vi "WFS Set Calc Spots To User Reference.vi"(7 "Array Ref Pos Y":u32, 8 "error in (no error)":errorcluster {"code" format="%.0x"}, 9 "Array Ref Pos X":u32, 10 "Reference Type (Relative)":i32(ring) items=["Relative", "Absolute"], 11 "instrument handle":refnum<visa-resource-name>) -> (0 "error out":errorcluster {"code" format="%.0x"}, 3 "instrument handle out":refnum<visa-resource-name>)   [LabVIEW 2020]
doc: "This VI sets the X and Y user reference spot positions in pixels to calculated spot positions given by two two-dimensional arrays."
uses:
  WFS_32.dll
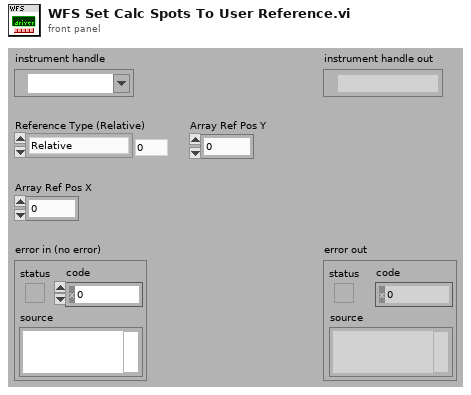
[diagram p1: front panel]
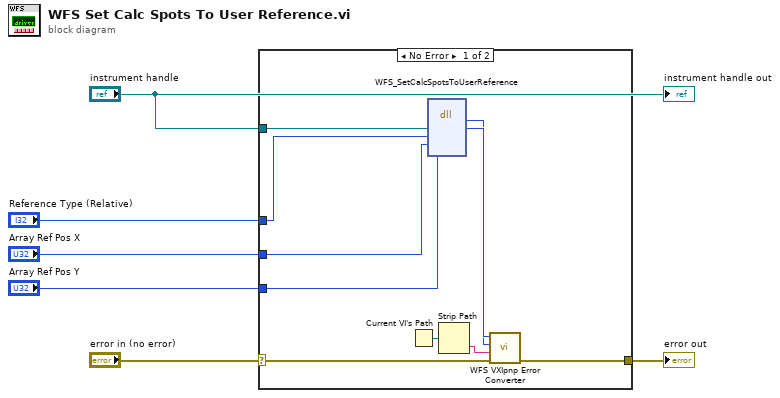
[diagram p0: block diagram]
diagram:
  n1 = case shown="No Error" "error in (no error)" {
    selector: "error in (no error)" -> [w11 w17]
    tunnel: [w10 w17] -> w6
    tunnel: "instrument handle" -> [w15 _]
    tunnel: "Reference Type (Relative)" -> [w9 _]
    tunnel: "Array Ref Pos X" -> [w8 _]
    tunnel: "Array Ref Pos Y" -> [w7 _]
    frame No Error {
      n2 = Current VI's Path() -> (path=w16:path)
      n3 = dll-call lib="WFS_*.*" fn="WFS_SetCalcSpotsToUserReference"("Instrument Handle"=w15, "Reference Type"=w9, "Array Ref Pos X"=w8, "Array Ref Pos Y"=w7) -> (w13:i32, "Instrument Handle"=w14:u32)  [unwired: 6 in, 2 out]
      n4 = Strip Path(path=w16) -> (name=w12:string)  [unwired: 1 out]
      n5 = call "WFS VXIpnp Error Converter.vi"("error in (no error)"=w11, "Name Of VI (\"\")"=w12, "CVI Error Code (0)"=w13, "instrument handle"=w14) -> ("error out"=w10:errorcluster)  [unwired: 6 in, 1 out]
    }
    frame Error {
    }
  }
  "error out" <- w6
  "instrument handle out" <- "instrument handle"
